vi "Reports.Station Configuration Report, Read or Write.vi"(8 "error in (no error)":errorcluster, 9 "Read(F)/Write(T)":bool, 10 "Test Result In":T1={"#attributes"={"Version"="MTE_1.0.0"}, "Facility"={"Name"="", "Location"=""}, "Station"={"Name"="", "PN"="", "SN"="", "Rev"="", "PC Name"="", "Location"="", "HW_Config"={"HW_Item"=[]}, "SW_Config"={"SW_Item"=[]}}, "Test Run"={"Operator"="", "Start Time"=timestamp(0 s since 1904-01-01), "Duration(s)"=0.0, "Mode"="", "Comment"="", "ProcessStep"=""}, "Test Sequence"={"Name"="", "Config"={"Config_Item"=[]}}, "UUTs"={"UUT"=[]}} {"UUTs"."UUT"."Attributes"."Attribute"."Status" items=["LOG", "PASS", "FAIL", "ERROR"]; "UUTs"."UUT"."Measurements"."Measurement"."Status" items=["LOG", "PASS", "FAIL", "ERROR"]}, 11 "Config Folder":path) -> (0 "error out":errorcluster, 2 "Test Result Out":T1={"#attributes"={"Version"="MTE_1.0.0"}, "Facility"={"Name"="", "Location"=""}, "Station"={"Name"="", "PN"="", "SN"="", "Rev"="", "PC Name"="", "Location"="", "HW_Config"={"HW_Item"=[]}, "SW_Config"={"SW_Item"=[]}}, "Test Run"={"Operator"="", "Start Time"=timestamp(0 s since 1904-01-01), "Duration(s)"=0.0, "Mode"="", "Comment"="", "ProcessStep"=""}, "Test Sequence"={"Name"="", "Config"={"Config_Item"=[]}}, "UUTs"={"UUT"=[]}} {"UUTs"."UUT"."Attributes"."Attribute"."Status" items=["LOG", "PASS", "FAIL", "ERROR"]; "UUTs"."UUT"."Measurements"."Measurement"."Status" items=["LOG", "PASS", "FAIL", "ERROR"]})   [LabVIEW 2018]
uses:
  Report.Result Report File Type.ctl
  Report.Result Report Config.ctl
  <vilib>/KATE/Files/File Utils.lvlib
  Results/Result XML/TestResult.HW Item.ctl
  Results/Result XML/TestResult.SW Item.ctl
  Results/Result XML/TestResult.Station Info.ctl
  Results/Result XML/TestResult.Test Run Info.ctl
  Results/Result XML/TestResult.Test Info.ctl
  Results/Result XML/TestResult.Symptom.State.ctl
  Results/Result XML/TestResult.Symptom.ctl
  Results/Result.Limit Type.ctl
  Results/Result.Measurement and Attribute Item Status.ctl
  Results/Result.Numeric.ctl
  Results/Result.Attribute.ctl
  Results/Result XML/TestResult.UUT Result.ctl
  Results/Result XML/TestResult.Facility.ctl
  Results/Result XML/TestResult.FullResultData.ctl
panel:
  out "JSON string":string
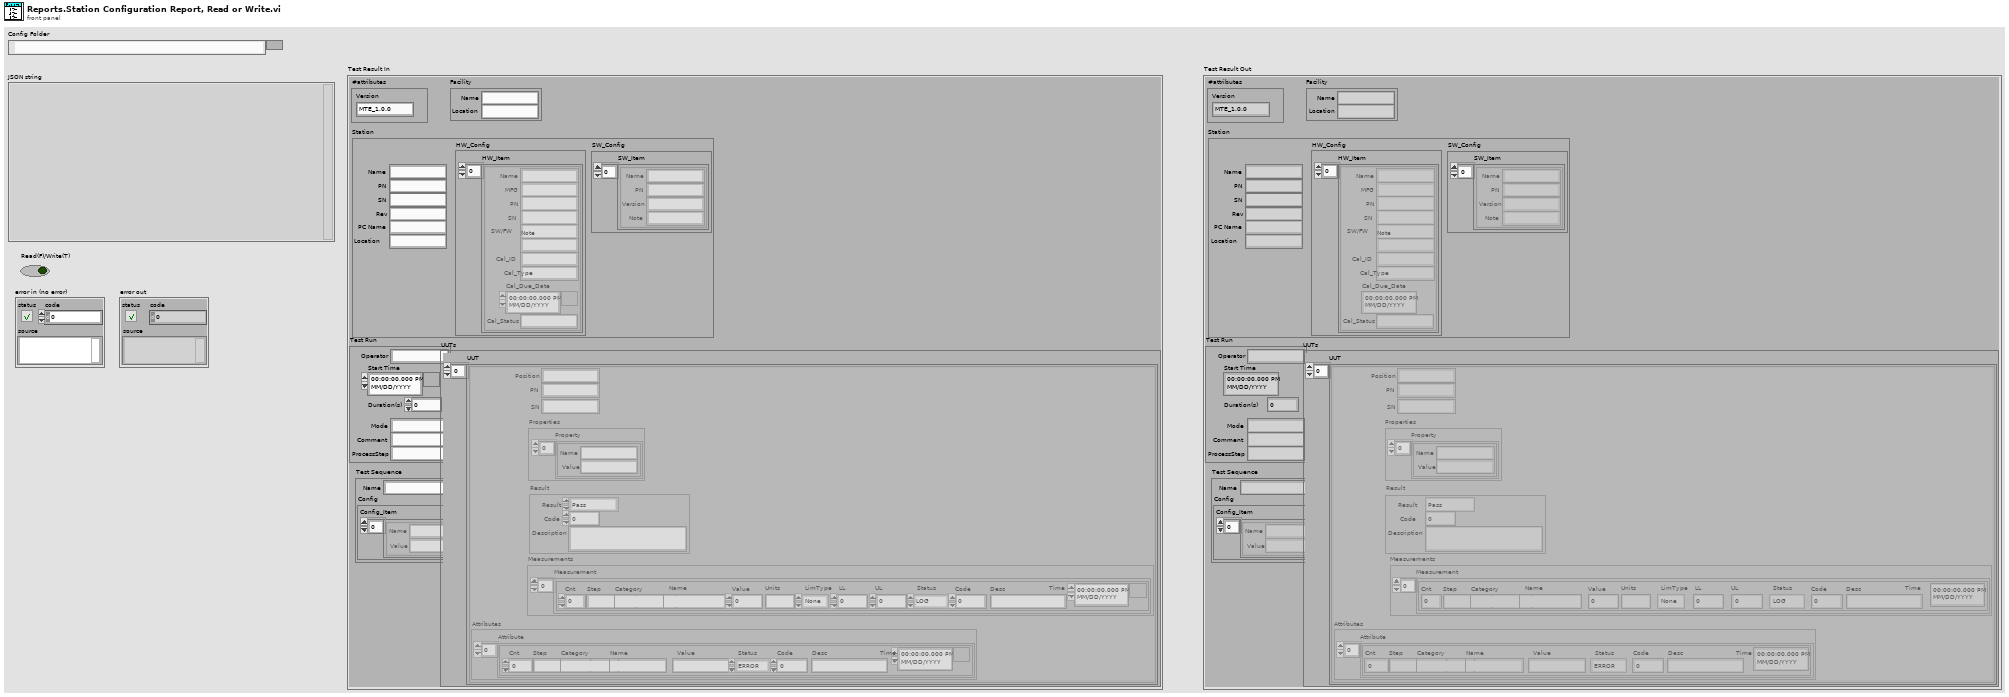
[diagram p1: front panel]
types:
  T1 = typedef "TestResult.FullResultData.ctl" = cluster{"#attributes":cluster{"Version":string}, "Facility":T2, "Station":T3, "Test Run":T6, "Test Sequence":T7, "UUTs":cluster{"UUT":T8[]}}
  T2 = typedef "TestResult.Facility.ctl" = cluster{"Name":string, "Location":string}
  T3 = typedef "TestResult.Station Info.ctl" = cluster{"Name":string, "PN":string, "SN":string, "Rev":string, "PC Name":string, "Location":string, "HW_Config":cluster{"HW_Item":T4[]}, "SW_Config":cluster{"SW_Item":T5[]}}
  T4 = typedef "TestResult.HW Item.ctl" = cluster{"Name":string, "MFG":string, "PN":string, "SN":string, "SW/FW":string, "Note":string, "Cal_ID":string, "Cal_Type":string, "Cal_Due_Date":timestamp, "Cal_Status":string}
  T5 = typedef "TestResult.SW Item.ctl" = cluster{"Name":string, "PN":string, "Version":string, "Note":string}
  T6 = typedef "TestResult.Test Run Info.ctl" = cluster{"Operator":string, "Start Time":timestamp, "Duration(s)":dbl, "Mode":string, "Comment":string, "ProcessStep":string}
  T7 = typedef "TestResult.Test Info.ctl" = cluster{"Name":string, "Config":cluster{"Config_Item":cluster{"Name":string, "Value":string}[]}}
  T8 = typedef "TestResult.UUT Info.ctl" = cluster{"Position":string, "PN":string, "SN":string, "Properties":cluster{"Property":cluster{"Name":string, "Value":string}[]}, "Result":T9, "Measurements":cluster{"Measurement":T11[]}, "Attributes":cluster{"Attribute":T14[]}}
  T9 = typedef "TestResult.Symptom.ctl" = cluster{"Result":T10, "Code":i32, "Description":string}
  T10 = typedef "TestResult.Symptom.State.ctl" = enum16{"Pass", "Fail", "Error", "Aborted", "Completed", "Logged"}
  T11 = typedef "Result.Numeric.ctl" = cluster{"Cnt":i32, "Step":string, "Category":string, "Name":string, "Value":dbl, "Units":string, "LimType":T12, "LL":dbl, "UL":dbl, "Status":T13, "Code":i32, "Desc":string, "Time":timestamp}
  T12 = typedef "Result.Limit Type.ctl" = enum16{"None", "EQ", "NE", "GT", "LT", "GE", "LE", "GTLT", "GELE", "GELT", "GTLE", "LTGT", "LEGE", "LEGT", "LTGE"}
  T13 = typedef "Result.Measurement and Attribute Item Status.ctl" = i32
  T14 = typedef "Result.Attribute.ctl" = cluster{"Cnt":i32, "Step":string, "Category":string, "Name":string, "Value":string, "Status":T13, "Code":i32, "Desc":string, "Time":timestamp}
  T15 = typedef "Report.Result Report File Type.ctl" = enum16{"Xlink", "XML_01", "XML_01_wFiles", "JSON_01", "JSON_01_wFiles"}
  T16 = typedef "Report.Result Report Config.ctl" = cluster{"Name":string, "Type":T15, "OutputDir":path}
  T17 = cluster{"Name":string, "Type":string, "Path":string}
  T18 = cluster{"Reports":cluster{"Name":string, "Type":string, "Path":string}[]}
  T19 = cluster{"Name":string, "Type":string, "Path":string}[]
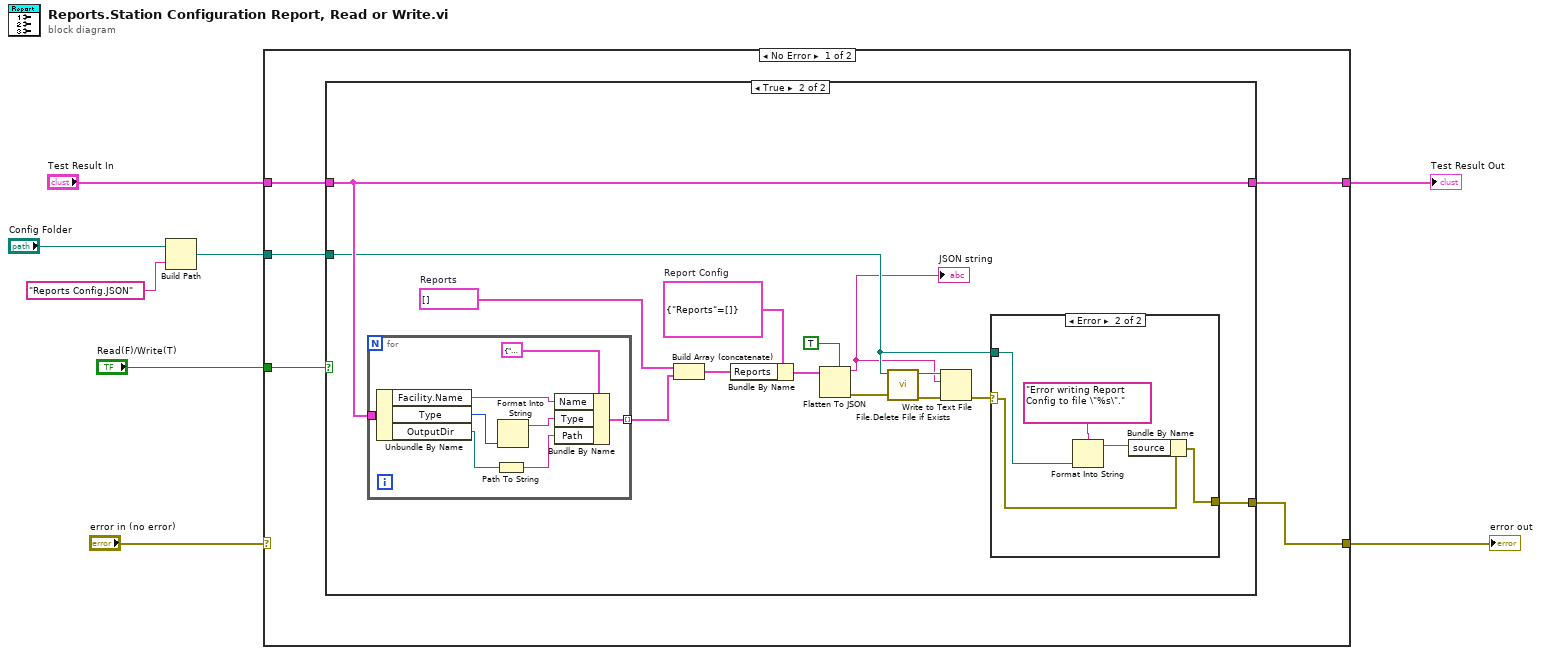
[diagram p0: block diagram]
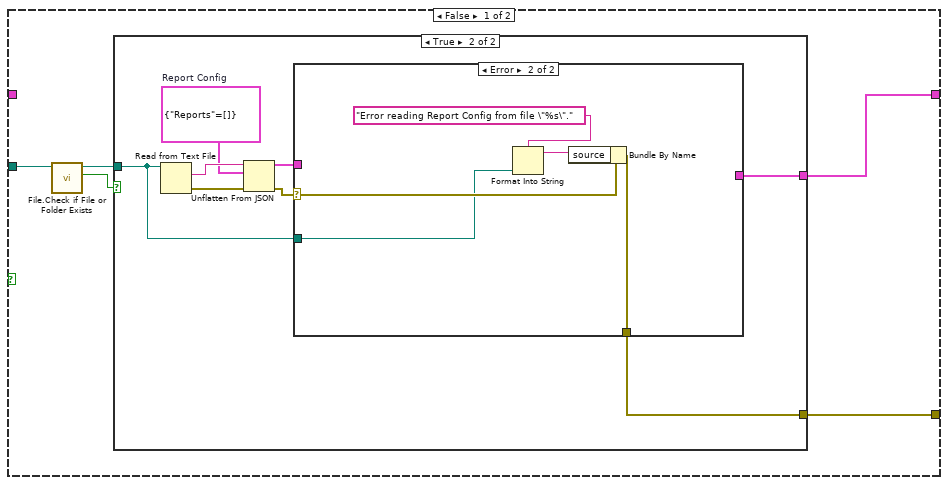
[diagram p2: hidden frame]
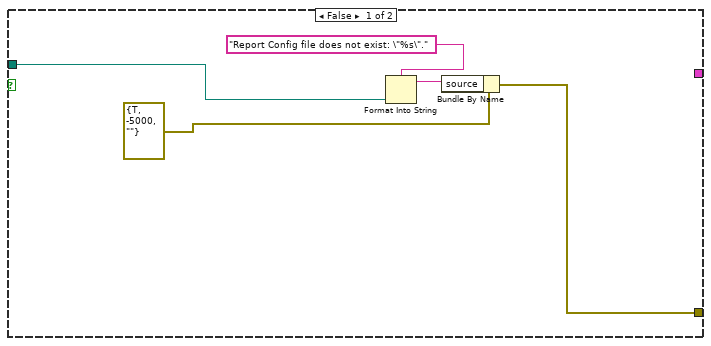
[diagram p3: hidden frame]
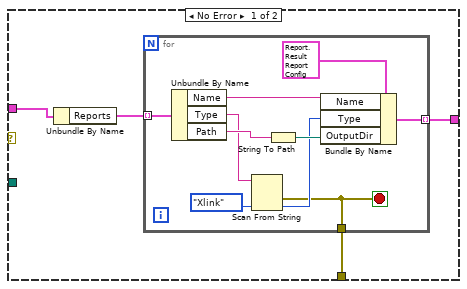
[diagram p4: hidden frame]
diagram:
  n1 = Build Path(base path="Config Folder", name or relative path="Reports Config.JSON") -> (appended path=w2:path)
  n2 = case shown="No Error" "error in (no error)" {
    selector: "error in (no error)" -> [_ w78]
    tunnel: "Read(F)/Write(T)" -> [w13 _]
    tunnel: "Test Result In" -> [w12 w79]
    tunnel: [w9 w79] -> w1
    tunnel: [w10 w78] -> w3
    tunnel: w2 -> [w11 _]
    frame No Error {
      n3 = case shown="True" w13 {
        tunnel: w12 -> [_ w62]
        tunnel: w11 -> [w16 w55]
        tunnel: [w17 w56] -> w10
        tunnel: [w18 w62] -> w9
        frame False {
          n4 = call <vilib>:"File.Check if File or Folder Exists.vi"("Path"=w16) -> ("Exists"=w14:bool, "Dup Path"=w15:path)  [unwired: 6 in, 3 out]
          n5 = case shown="True" w14 {
            tunnel: [_ w29] -> w18
            tunnel: [w19 w28] -> w17
            tunnel: w15 -> [w20 w24]
            frame False {
              n6 = Format Into String(format string="Report Config file does not exist: \"%s\".", w20) -> (resulting string=w23:string)  [unwired: 2 in, 1 out]
              n7 = Bundle By Name(cluster=errorcluster {"status"=TRUE, "code"=-5000, "source"=""} ("error constant"), "source"=w23) -> (w19:errorcluster)
            }
            frame True {
              w25 = T18 {"Reports"=[]}  # Report Config
              n8 = Read from Text File(file (use dialog)=w24) -> (text=w31:string, error out=w26:errorcluster)  [unwired: 3 in, 2 out]
              n9 = Unflatten From JSON(JSON string=w31, type and defaults=w25, error in (no error)=w26) -> (value=w30:T18, error out=w27:errorcluster)  [unwired: 4 in]
              n10 = case shown="Error" w27 {
                selector: w27 -> [_ w50]
                tunnel: w30 -> [w33 _]
                tunnel: [w35 _] -> w29
                tunnel: [w34 w49] -> w28
                tunnel: w24 -> [_ w46]
                frame No Error {
                  n11 = Unbundle By Name(w33) -> ("Reports"=w32:T19)
                  n12 = for {
                    tunnel: w32 -> [w45] mode=indexing
                    tunnel: [w41] -> w35 mode=indexing
                    tunnel: [w36] -> w34
                    stop <- w36 stop-if-true
                    n13 = Unbundle By Name(w45) -> ("Name"=w43:string, "Type"=w39:string, "Path"=w44:string)
                    n14 = Scan From String(input string=w39, default 1=Report.Result_Report_File_Type."Xlink" ("Type")) -> (error out=w36:errorcluster, output 1=w37:T15)  [unwired: 3 in, 2 out]
                    n15 = String To Path(string=w44) -> (path=w42:path)
                    n16 = Bundle By Name(cluster=T16 {"Name"="", "Type"=enum."JSON_01_wFiles", "OutputDir"=path ""} ("Report Config In"), "Name"=w43, "Type"=w37, "OutputDir"=w42) -> (w41:T16)
                  }
                }
                frame Error {
                  n17 = Format Into String(format string="Error reading Report Config from file \"%s\".", w46) -> (resulting string=w48:string)  [unwired: 2 in, 1 out]
                  n18 = Bundle By Name(cluster=w50, "source"=w48) -> (w49:errorcluster)
                }
              }
            }
          }
        }
        frame True {
          w59 = T18 {"Reports"=[]}  # Report Config
          w60 = T19 []  # Reports
          n19 = for {
            tunnel: w62 -> [w77]
            tunnel: [w70] -> w61 mode=indexing
            n20 = Unbundle By Name(w77) -> ("Facility.Name"=w73:string, "Type"=w76:T15, "OutputDir"=w75:path)
            n21 = Path To String(path=w75) -> (string=w71:string)
            n22 = Format Into String(w76) -> (resulting string=w72:string)  [unwired: 3 in, 1 out]
            n23 = Bundle By Name(cluster=T17 {"Name"="", "Type"="", "Path"=""} ("Report"), "Name"=w73, "Type"=w72, "Path"=w71) -> (w70:T17)
          }
          n24 = Build Array (concatenate)(w60, w61) -> (w58:T19)
          n25 = Bundle By Name(cluster=w59, "Reports"=w58) -> (w57:T18)
          n26 = Flatten To JSON(enable LabVIEW extensions? (T)=TRUE, anything=w57) -> (JSON string=w51:string, 11:w63:errorcluster)  [unwired: 1 in]
          "JSON string" <- w51
          n27 = call "File.Delete File if Exists.vi"("error in"=w63, "Path"=w55) -> ("error out"=w54:errorcluster, "Path Out"=w53:path)  [unwired: 8 in]
          n28 = Write to Text File(file (use dialog)=w53, text=w51, error in=w54) -> (error out=w52:errorcluster)  [unwired: 1 in, 2 out]
          n29 = case shown="Error" w52 {
            selector: w52 -> [_ w67]
            tunnel: [_ w66] -> w56
            tunnel: w55 -> [_ w65]
            frame No Error {
            }
            frame Error {
              n30 = Format Into String(format string="Error writing Report Config to file \"%s\".", w65) -> (resulting string=w69:string)  [unwired: 2 in, 1 out]
              n31 = Bundle By Name(cluster=w67, "source"=w69) -> (w66:errorcluster)
            }
          }
        }
      }
    }
    frame Error {
    }
  }
  "error out" <- w3
  "Test Result Out" <- w1
